vi "A87.6-encoder.vi"(10 "参考电压Vref（V）":dbl=2.56, 11 "信号数组":dbl[](array[numeric])) -> (3 "编码数组":digitaldata)   [LabVIEW 2018]
uses:
  <vilib>/Waveform/DWDTOps.llb/DWDT Binary U8 to Digital.vi
panel:
  # "输入：信号数组，参考电压Vref\n输出：编码数组（数字数据）"
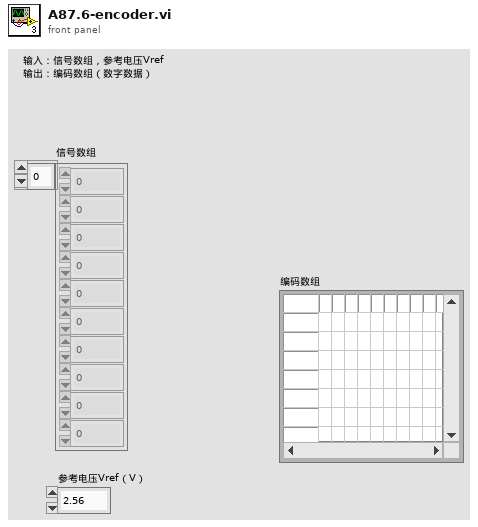
[diagram p1: front panel]
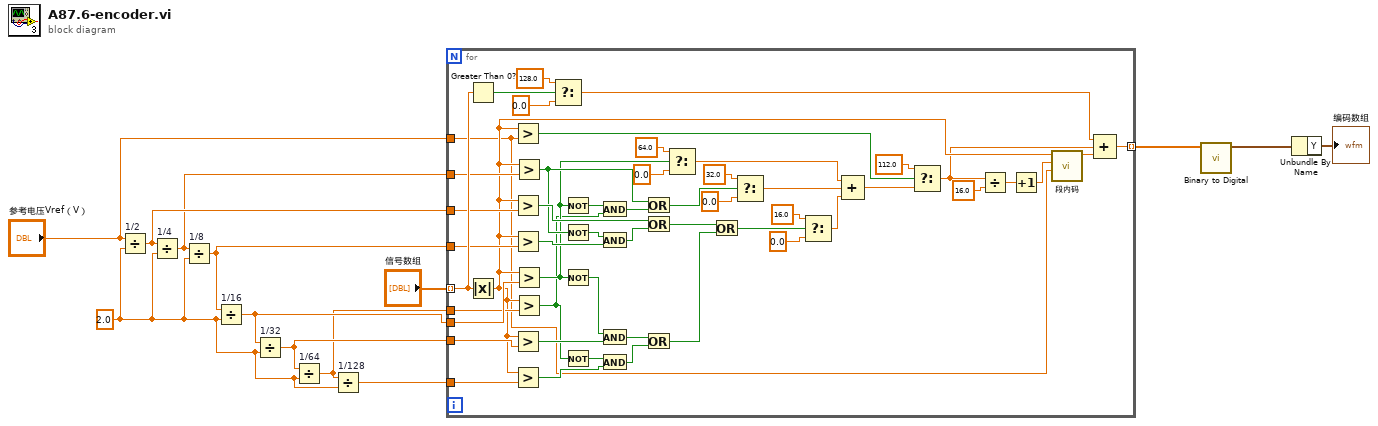
[diagram p0: block diagram]
diagram:
  w7 = 2.0 ("y")
  n1 = Divide "1/2"(x="参考电压Vref（V）", y=w7) -> (x/y=w12:dbl)
  n2 = Divide "1/4"(x=w12, y=w7) -> (x/y=w11:dbl)
  n3 = Divide "1/8"(x=w11, y=w7) -> (x/y=w10:dbl)
  n4 = Divide "1/16"(x=w10, y=w7) -> (x/y=w9:dbl)
  n5 = Divide "1/32"(x=w9, y=w7) -> (x/y=w8:dbl)
  n6 = Divide "1/64"(x=w8, y=w7) -> (x/y=w6:dbl)
  n7 = Divide "1/128"(x=w6, y=w7) -> (x/y=w5:dbl)
  n8 = for {
    tunnel: "信号数组" -> [w63] mode=indexing
    tunnel: w12 -> [w58]
    tunnel: w11 -> [w57]
    tunnel: w10 -> [w56]
    tunnel: w9 -> [w55]
    tunnel: w8 -> [w54]
    tunnel: w6 -> [w53]
    tunnel: w5 -> [w52]
    tunnel: "参考电压Vref（V）" -> [w17]
    tunnel: [w22] -> w3 mode=indexing
    n9 = Greater Than 0?(x=w63) -> (x > 0?=w64:bool)
    n10 = Absolute Value(x=w63) -> (abs(x)=w18:dbl)
    n11 = Greater?(x=w18, y=w17) -> (0:w16:bool)
    n12 = Greater?(x=w18, y=w58) -> (0:w44:bool)
    n13 = Greater?(x=w18, y=w56) -> (0:w41:bool)
    n14 = Greater?(x=w18, y=w54) -> (0:w37:bool)
    n15 = Greater?(x=w18, y=w52) -> (0:w34:bool)
    n16 = Greater?(x=w18, y=w57) -> (0:w42:bool)
    n17 = Greater?(x=w18, y=w55) -> (0:w38:bool)
    n18 = Greater?(x=w18, y=w53) -> (0:w35:bool)
    n19 = Select(t=128.0, s=w64, f=0.0) -> (s? t:f=w24:dbl)
    n20 = Not(x=w38) -> (.not. x?=w47:bool)
    n21 = Not(x=w42) -> (.not. x?=w43:bool)
    n22 = Not(x=w38) -> (.not. x?=w39:bool)
    n23 = Not(x=w35) -> (.not. x?=w36:bool)
    n24 = And(x=w47, y=w35) -> (x .and. y?=w46:bool)
    n25 = And(x=w43, y=w41) -> (x .and. y?=w40:bool)
    n26 = And(x=w39, y=w37) -> (x .and. y?=w33:bool)
    n27 = And(x=w36, y=w34) -> (x .and. y?=w32:bool)
    n28 = Or(x=w42, y=w46) -> (x .or. y?=w45:bool)
    n29 = Or(x=w44, y=w40) -> (x .or. y?=w31:bool)
    n30 = Or(x=w33, y=w32) -> (x .or. y?=w30:bool)
    n31 = Select(t=64.0, s=w38, f=0.0) -> (s? t:f=w28:dbl)
    n32 = Or(x=w31, y=w30) -> (x .or. y?=w29:bool)
    n33 = Select(t=32.0, s=w45, f=0.0) -> (s? t:f=w27:dbl)
    n34 = Select(t=16.0, s=w29, f=0.0) -> (s? t:f=w26:dbl)
    n35 = Compound Arithmetic op=ADD(w28, w27, w26) -> (w19:dbl)
    n36 = Select(t=112.0, s=w16, f=w19) -> (s? t:f=w15:dbl)
    n37 = Divide(x=w15, y=16.0) -> (x/y=w21:dbl)
    n38 = Increment(x=w21) -> (x+1=w20:dbl)
    n39 = call "段内码.vi"("参考电压（V）"=w17, "段落位置"=w20, "信号电压"=w18) -> ("段内码"=w23:ext)  [unwired: 8 in]
    n40 = Compound Arithmetic op=ADD(w24, w15, w23) -> (w22:ext)
  }
  n41 = call-poly <vilib>:"Binary to Digital.vi"("binary array"=w3) -> ("digital waveform"=w2:digitalwaveform)  [unwired: 9 in, 1 out]
  n42 = Unbundle By Name ("获取波形成分")(w2) -> ("Y"=→"编码数组":digitaldata)
